vi "Flatten.vi"(6 "Persistence in":refnum<class "IPersist.lvclass">, 7 "Linked List Ref":refnum<data-value>, 8 "error in (no error)":errorcluster, 9 "Indent":i32, 10 "Active Unique ID":string, 11 "Loop in":refnum<class "Loop.lvclass">) -> (0 "error out":errorcluster, 2 "Active Unique ID out":string, 3 "Flattened Test Executive":string[](array[string]), 4 "Persistence out":refnum<class "IPersist.lvclass">, 5 "Linked List Ref out":refnum<data-value>)   [LabVIEW 2020, in "Test Executive.lvlib" / "Loop.lvclass"]
uses:
  <vilib>/gpm_packages/@cs/test-executive/Source/Test Executive/Loop/Loop.lvclass
  <vilib>/gpm_packages/@cs/linked-list/Source/Linked List/ILinkedList/ILinked List.lvclass
  <vilib>/gpm_packages/@cs/persistence/source/IPersist/IPersist.lvclass
  <vilib>/gpm_packages/@cs/test-executive/Source/Test Executive/Executioner/Executioner.lvclass
  <vilib>/gpm_packages/@cs/linked-list/Source/Linked List/Linked List Ref/Linked List Ref.lvclass
  <vilib>/gpm_packages/@cs/linked-list/Source/String Manipulation/String Manipulation.lvlib
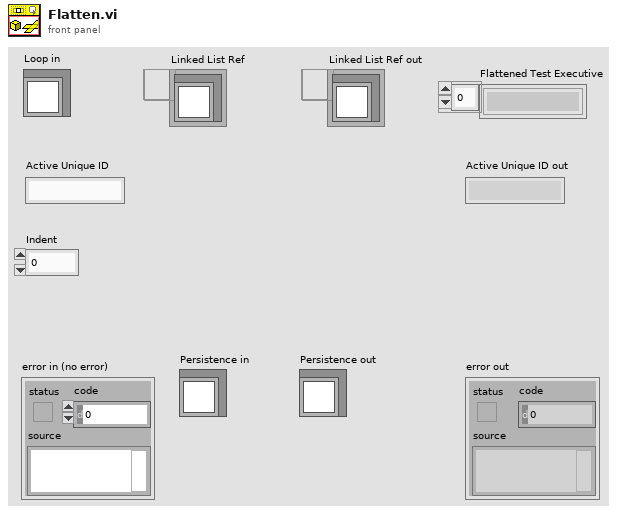
[diagram p1: front panel]
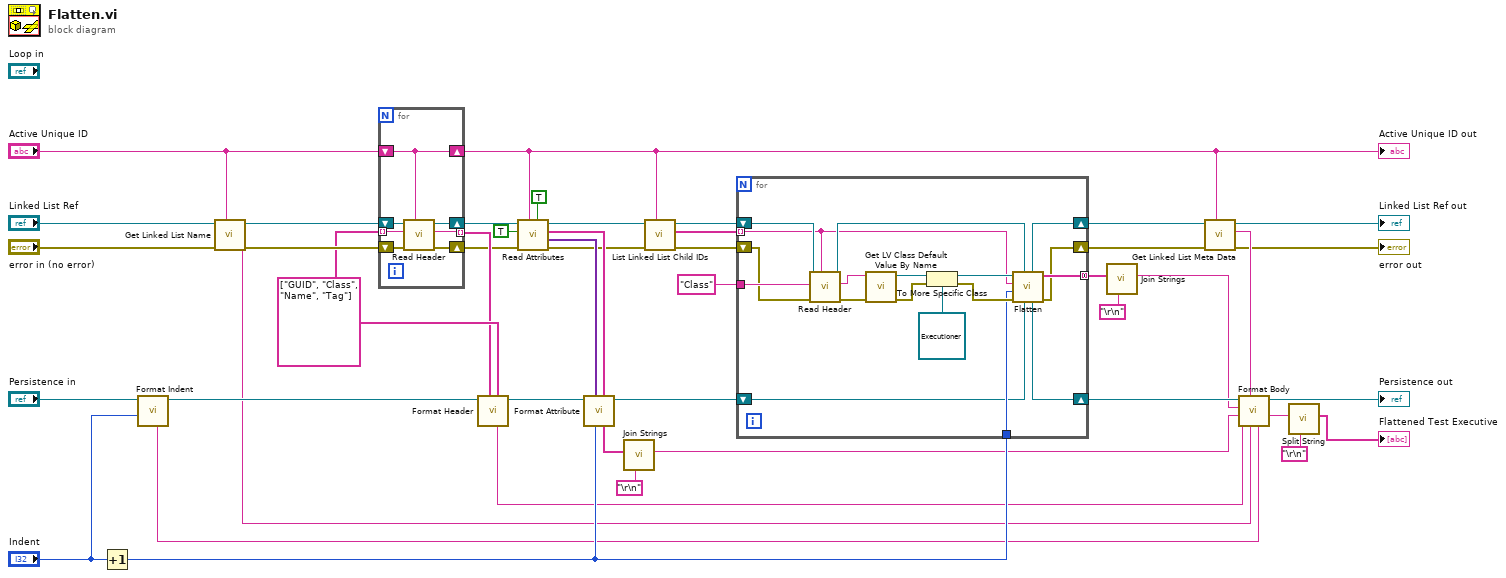
[diagram p0: block diagram]
diagram:
  w38 = string[] ["GUID", "Class", "Name", "Tag"] ("Header Names")
  n1 = Increment(x="Indent") -> (x+1=w18:i32)
  n2 = call-dynamic "Format Indent.vi"("Indent"="Indent", "IPersist in"="Persistence in") -> ("IPersist out"=w39:refnum<class "IPersist.lvclass">, "Indent XML"=w4:string)  [unwired: 7 in, 1 out]
  n3 = call <vilib>:"Get Linked List Name.vi"("Linked List ID"="Active Unique ID", "error in (no error)"="error in (no error)", "Linked List Ref"="Linked List Ref") -> ("error out"=w41:errorcluster, "Linked List Name"=w5:string, "Linked List Ref out"=w42:refnum<data-value>)  [unwired: 5 in, 1 out]
  n4 = for {
    tunnel: w38 -> [w50] mode=indexing
    shift-right: [w51] -> w31
    shift-left: w42 -> [w52]
    tunnel: [w49] -> w37 mode=indexing
    shift-right: [w48] -> w12
    shift-left: "Active Unique ID" -> [w48]
    shift-right: [w46] -> w30
    shift-left: w41 -> [w47]
    n5 = call <vilib>:"Read Header.vi"("Linked List ID"=w48, "error in (no error)"=w47, "Header Name"=w50, "Linked List Ref"=w52) -> ("error out"=w46:errorcluster, "Header Value"=w49:string, "Linked List Ref out"=w51:refnum<data-value>)  [unwired: 4 in, 1 out]
  }
  "Active Unique ID out" <- w12
  n6 = call-dynamic "Format Header.vi"("Name"=w38, "Value"=w37, "IPersist in"=w39) -> ("IPersist out"=w29:refnum<class "IPersist.lvclass">, "Header"=w6:string)  [unwired: 7 in]
  n7 = call <vilib>:"Read Attributes.vi"("Flatten Pointer?"=TRUE, "Linked List ID"=w12, "error in (no error)"=w30, "Include Private?"=TRUE, "Linked List Ref"=w31) -> ("error out"=w26:errorcluster, "Attributes"=w35:variant[], "Attribute Names out"=w34:string[], "Linked List Ref out"=w27:refnum<data-value>)  [unwired: 1 in, 2 out]
  n8 = call-dynamic "Format Attribute.vi"("Attribute Names"=w34, "Indent"=w18, "Attribute Values"=w35, "IPersist in"=w29) -> ("IPersist out"=w19:refnum<class "IPersist.lvclass">, "Attr Strings"=w32:string[])  [unwired: 6 in]
  n9 = call <vilib>:"Join Strings.vi"("Separator (,)"="\r\n", "Strings In"=w32) -> ("String"=w7:string)  [unwired: 9 in]
  n10 = call <vilib>:"List Linked List Child IDs.vi"("Linked List ID"=w12, "error in (no error)"=w26, "Linked List Ref"=w27) -> ("error out"=w21:errorcluster, "Child IDs"=w20:string[], "Linked List Ref out"=w22:refnum<data-value>)  [unwired: 6 in]
  n11 = for {
    shift-right: [w70] -> w3
    shift-left: w22 -> [w69]
    tunnel: w20 -> [w57] mode=indexing
    tunnel: w18 -> [w60]
    shift-right: [w58] -> w14
    shift-left: w19 -> [w59]
    tunnel: [w56] -> w24 mode=concatenating
    shift-right: [w53] -> w2
    shift-left: w21 -> [w54]
    tunnel: "Class" ("Header Name") -> [w55]
    n12 = call <vilib>:"Read Header.vi"("Linked List ID"=w57, "error in (no error)"=w54, "Header Name"=w55, "Linked List Ref"=w69) -> ("error out"=w63:errorcluster, "Header Value"=w64:string, "Linked List Ref out"=w68:refnum<data-value>)  [unwired: 4 in, 1 out]
    n13 = call <vilib>:"Get LV Class Default Value By Name.vi"("error in (no error)"=w63, "class name"=w64) -> ("error out"=w65:errorcluster, "object"=w67:refnum<class>)  [unwired: 8 in]
    n14 = To More Specific Class(target class=refnum<class "Executioner.lvclass"> refnum ("Test Executive.lvlib:Executioner.lvclass"), reference=w67, error in=w65) -> (specific class reference=w62:refnum<class "Executioner.lvclass">, error out=w61:errorcluster)
    n15 = call-dynamic "Flatten.vi"("Persistence in"=w59, "Linked List Ref"=w68, "error in (no error)"=w61, "Indent"=w60, "Active Unique ID"=w57, "Executioner in"=w62) -> ("error out"=w53:errorcluster, "Flattened Test Executive"=w56:string[], "Persistence out"=w58:refnum<class "IPersist.lvclass">, "Linked List Ref out"=w70:refnum<data-value>)  [unwired: 1 in, 1 out]
  }
  n16 = call <vilib>:"Join Strings.vi"("Separator (,)"="\r\n", "Strings In"=w24) -> ("String"=w13:string)  [unwired: 9 in]
  n17 = call <vilib>:"Get Linked List Meta Data.vi"("Linked List ID"=w12, "error in (no error)"=w2, "Linked List Ref"=w3) -> ("error out"=→"error out":errorcluster, "Meta Data"=w17:string, "Linked List Ref out"=→"Linked List Ref out":refnum<data-value>)  [unwired: 5 in, 1 out]
  n18 = call-dynamic "Format Body.vi"("Indent"=w4, "Name"=w5, "Meta Data"=w17, "Header"=w6, "Attributes"=w7, "Body"=w13, "IPersist in"=w14) -> ("String out"=w15:string, "IPersist out"=→"Persistence out":refnum<class "IPersist.lvclass">)  [unwired: 3 in]
  n19 = call <vilib>:"Split String.vi"("Split Pattern"="\r\n", "Input String"=w15) -> ("Split String"=→"Flattened Test Executive":string[])  [unwired: 9 in]
